vi "2 WaypointHeadingGoodness.vi"(4 "Heading to Test":dbl) -> (1 "Goodness":dbl)   [LabVIEW 2011]
doc: "Takes the absolute wind vector, the heading of your next waypoint, and your current heading, and recommends a heading.\n\nWe repeatedly run the iterate theta VI until its outputs converge. The converging outputs are the two angles which minimize the travel time to the waypoint.\n\nAfter the while loop, we determine which angle is closer to the current heading. We choose the closer heading unless the other heading has a significantly higher dr/dt."
uses:
  2 Globals/2 Global.vi
  2 Classes/Waypoint/Waypoint.lvclass
panel:
  in  "Waypoint East":dbl
  in  "Waypoint North":dbl
  in  "Wind Angle":dbl
  # "Inputs"
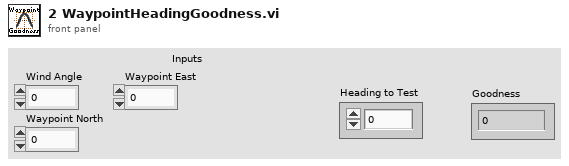
[diagram p1: front panel]
types:
  T1 = typedef "Velocity.ctl" = cluster{"East":dbl, "North":dbl}
  T2 = typedef "UTM Location.ctl" = cluster{"UTM Zone":dbl, "Hemisphere":enum16{"North", "South"}, "East":dbl, "North":dbl}
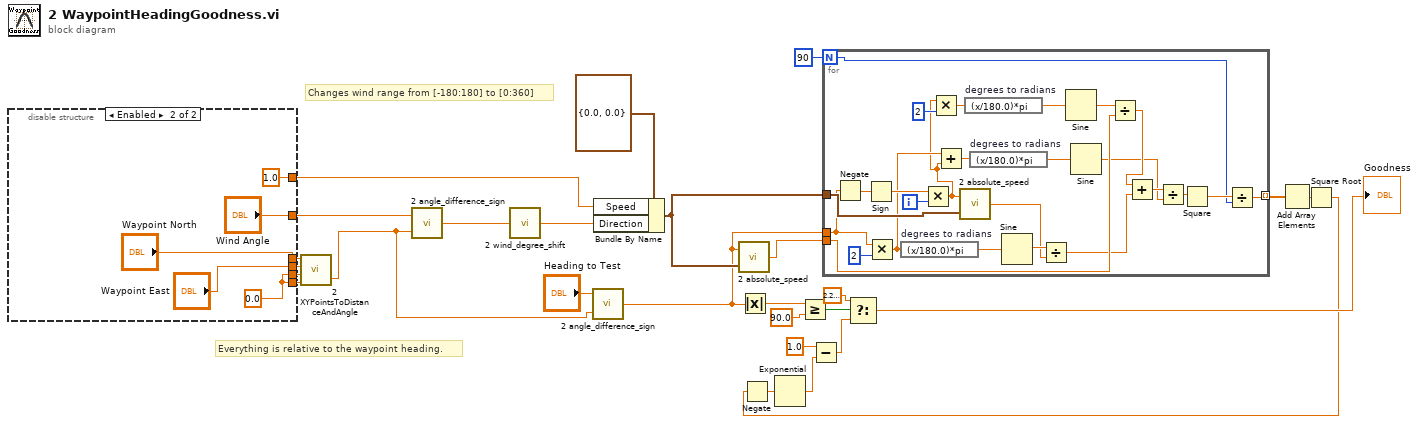
[diagram p0: block diagram]
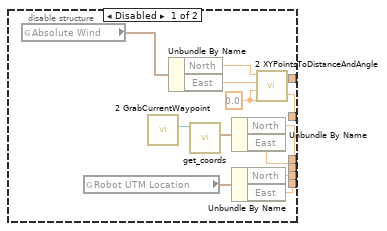
[diagram p2: hidden frame]
diagram:
  # "Changes wind range from [-180:180] to [0:360]"
  # "Everything is relative to the waypoint heading."
  n1 = disable-structure shown="Enabled" {
    disable-tunnel: [w33 "Wind Angle"] -> w6
    disable-tunnel: [w32 1.0 ("Distance")] -> w5
    disable-tunnel: [w31 w43] -> w4
    disable-tunnel: [w30 w43] -> w3
    disable-tunnel: [w29 "Waypoint North"] -> w2
    disable-tunnel: [w28 "Waypoint East"] -> w1
    frame Disabled {
      w34 = 0.0
      n2 = global read "2 Global.vi" "Absolute Wind"() -> (w37:T1)
      n3 = global read "2 Global.vi" "Robot UTM Location"() -> (w38:T2)
      n4 = call "2 GrabCurrentWaypoint.vi"() -> ("Current Waypoint"=w40:refnum<class "Waypoint.lvclass">)  [unwired: 11 in]
      n5 = Unbundle By Name(w37) -> ("North"=w35:dbl, "East"=w36:dbl)
      n6 = call-dynamic "get_coords.vi"("Waypoint in"=w40) -> ("Coords"=w39:T2)  [unwired: 7 in, 3 out]
      n7 = Unbundle By Name(w39) -> ("North"=w29:dbl, "East"=w28:dbl)
      n8 = Unbundle By Name(w38) -> ("North"=w30:dbl, "East"=w31:dbl)
      n9 = call "2 XYPointsToDistanceAndAngle.vi"("East 2"=w34, "North 2"=w34, "East 1"=w36, "North 1"=w35) -> ("Angle Diff"=w33:dbl, "Distance"=w32:dbl)
    }
    frame Enabled {
      w43 = 0.0 ("Distance")
    }
  }
  n10 = call "2 XYPointsToDistanceAndAngle.vi"("East 2"=w4, "North 2"=w3, "East 1"=w1, "North 1"=w2) -> ("Angle Diff"=w23:dbl)  [unwired: 1 out]
  n11 = call "2 angle_difference_sign.vi"("Angle 2"=w23, "Angle 1"=w6) -> ("Difference"=w27:dbl)
  n12 = call "2 wind_degree_shift.vi"("Wind Theta -180 - 180"=w27) -> ("Wind Theta 0-360"=w26:dbl)
  n13 = call "2 angle_difference_sign.vi"("Angle 2"=w23, "Angle 1"="Heading to Test") -> ("Difference"=w11:dbl)
  n14 = Bundle By Name(cluster=cluster{"Speed":dbl, "Direction":dbl} {"Speed"=0.0, "Direction"=0.0} ("input cluster"), "Speed"=w5, "Direction"=w26) -> (w12:cluster{"Speed":dbl, "Direction":dbl})
  n15 = call "2 absolute_speed.vi"("Wind Vector"=w12, "Boat Angle"=w11) -> ("Velocity"=w13:dbl)
  n16 = Absolute Value(x=w11) -> (abs(x)=w19:dbl)
  n17 = Greater Or Equal?(x=w19, y=90.0) -> (x >= y?=w21:bool)
  n18 = for {
    N: 90 -> [w46]
    tunnel: w13 -> [w56]
    tunnel: w12 -> [w71]
    tunnel: w11 -> [w65]
    tunnel: [w48] -> w10 mode=indexing
    i -> [w70]
    n19 = Negate(x=w65) -> (-x=w68:dbl)
    n20 = Sign(1:w68) -> (0:w69:dbl)
    n21 = Multiply(x=w65, y=2) -> (x*y=w62:dbl)
    n22 = expression code="(x/180.0)*pi" "degrees to radians"(w62) -> (w67:dbl)
    n23 = Multiply(x=w69, y=w70) -> (x*y=w58:dbl)
    n24 = Multiply(x=w58, y=2) -> (x*y=w61:dbl)
    n25 = Add(x=w62, y=w58) -> (x+y=w63:dbl)
    n26 = call "2 absolute_speed.vi"("Wind Vector"=w71, "Boat Angle"=w58) -> ("Velocity"=w54:dbl)
    n27 = expression code="(x/180.0)*pi" "degrees to radians"(w61) -> (w59:dbl)
    n28 = expression code="(x/180.0)*pi" "degrees to radians"(w63) -> (w64:dbl)
    n29 = Sine(x=w67) -> (sin(x)=w55:dbl)
    n30 = Divide(x=w55, y=w54) -> (x/y=w52:dbl)
    n31 = Sine(x=w59) -> (sin(x)=w57:dbl)
    n32 = Sine(x=w64) -> (sin(x)=w50:dbl)
    n33 = Divide(x=w57, y=w56) -> (x/y=w53:dbl)
    n34 = Add(x=w53, y=w52) -> (x+y=w51:dbl)
    n35 = Divide(x=w51, y=w50) -> (x/y=w49:dbl)
    n36 = Square(x=w49) -> (x^2=w47:dbl)
    n37 = Divide(x=w47, y=w46) -> (x/y=w48:dbl)
  }
  n38 = Add Array Elements(numeric array=w10) -> (sum=w8:dbl)
  n39 = Square Root(x=w8) -> (sqrt(x)=w7:dbl)
  n40 = Negate(x=w7) -> (-x=w15:dbl)
  n41 = Exponential(1:w15) -> (0:w16:dbl)
  n42 = Subtract(x=1.0, y=w16) -> (x-y=w14:dbl)
  n43 = Select(t=2.220446049250313e-16, s=w21, f=w14) -> (s? t:f=→"Goodness":dbl)
